vi "Refactor Object for Library Rename.vi"(8 "error in (no error)":errorcluster, 10 "rename data":T2, 11 "object reference in":refnum<vi>) -> (0 "error out":errorcluster, 1 "refactored dependency":bool, 2 "refactor result":T1, 3 "object reference out":refnum<vi>)   [LabVIEW 2020, in "MeasurementService Editor.lvlib"]
uses:
  MeasurementService Editor.lvlib
  Rename Refactor Data.ctl
  Rename Refactor Mapping Info.ctl
  Rename Refactor Result.ctl
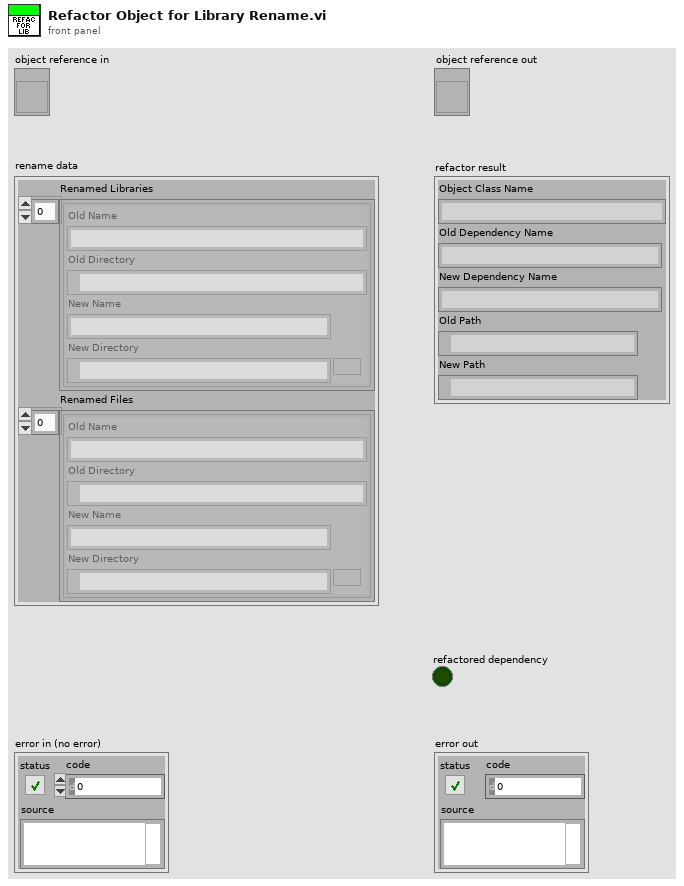
[diagram p1: front panel]
types:
  T1 = typedef "MeasurementService Editor.lvlib/Rename Refactor Result.ctl" = cluster{"Object Class Name":string, "Old Dependency Name":string, "New Dependency Name":string, "Old Path":path, "New Path":path}
  T2 = typedef "MeasurementService Editor.lvlib/Rename Refactor Data.ctl" = cluster{"Renamed Libraries":T3[], "Renamed Files":T3[]}
  T3 = typedef "MeasurementService Editor.lvlib/Rename Refactor Mapping Info.ctl" = cluster{"Old Name":string, "Old Directory":path, "New Name":string, "New Directory":path}
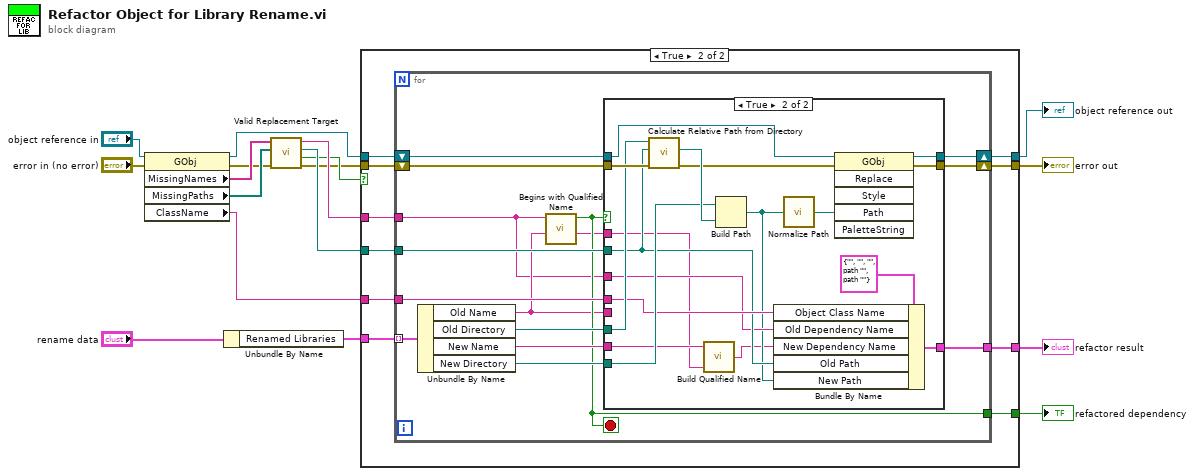
[diagram p0: block diagram]
diagram:
  n1 = property class="GObj"(reference="object reference in", error in="error in (no error)") -> (reference out=w8:refnum<vi>, error out=w2:errorcluster, "MissingNames"=w7:string[], "MissingPaths"=w6:path[], "ClassName"=w15:string)
  n2 = Unbundle By Name("rename data") -> ("Renamed Libraries"=w14:T3[])
  n3 = call "Valid Replacement Target.vi"("error in (no error)"=w2, "missing paths"=w6, "missing names"=w7) -> ("error out"=w1:errorcluster, "valid replacement target"=w3:bool, "missing path"=w4:path, "missing name"=w5:string)  [unwired: 5 in]
  n4 = case shown="True" w3 {
    tunnel: w8 -> [w18 w29]
    tunnel: w1 -> [w19 w28]
    tunnel: w5 -> [_ w20]
    tunnel: [w19 w23] -> w10
    tunnel: [w18 w24] -> w9
    tunnel: w15 -> [_ w25]
    tunnel: w4 -> [_ w26]
    tunnel: w14 -> [_ w27]
    tunnel: [_ w22] -> w12
    tunnel: [_ w21] -> w11
    frame False {
    }
    frame True {
      n5 = for {
        shift-right: [w40] -> w23
        shift-left: w28 -> [w42]
        shift-right: [w41] -> w24
        shift-left: w29 -> [w43]
        tunnel: w27 -> [w44] mode=indexing
        tunnel: w26 -> [w38]
        tunnel: [w33] -> w22
        tunnel: w25 -> [w36]
        tunnel: [w34] -> w21
        tunnel: w20 -> [w30]
        stop <- w33 stop-if-true
        n6 = Unbundle By Name(w44) -> ("Old Name"=w32:string, "Old Directory"=w39:path, "New Name"=w35:string, "New Directory"=w37:path)
        n7 = call "Begins with Qualified Name.vi"("beginning name"=w32, "name"=w30) -> ("ending name"=w31:string, "begins with name"=w33:bool)  [unwired: 8 in]
        n8 = case shown="True" w33 {
          tunnel: w43 -> [w46 w57]
          tunnel: w42 -> [w45 w64]
          tunnel: [w46 w58] -> w41
          tunnel: [w45 w60] -> w40
          tunnel: w39 -> [_ w63]
          tunnel: w38 -> [_ w54]
          tunnel: w37 -> [_ w61]
          tunnel: w36 -> [_ w55]
          tunnel: w32 -> [_ _]
          tunnel: w35 -> [_ w49]
          tunnel: [_ w53] -> w34
          tunnel: w31 -> [_ w48]
          tunnel: w30 -> [_ w52]
          frame False {
          }
          frame True {
            n9 = call "Calculate Relative Path from Directory.vi"("error in (no error)"=w64, "path"=w54, "directory"=w63) -> ("error out"=w59:errorcluster, "relative path"=w62:path)  [unwired: 7 in]
            n10 = call "Build Qualified Name.vi"("name"=w48, "base name"=w49) -> ("appended name"=w47:string)  [unwired: 3 in]
            n11 = Build Path(base path=w61, name or relative path=w62) -> (appended path=w51:path)
            n12 = Bundle By Name(cluster=T1 {"Object Class Name"="", "Old Dependency Name"="", "New Dependency Name"="", "Old Path"=path "", "New Path"=path ""} ("Rename Refactor Result"), "Object Class Name"=w55, "Old Dependency Name"=w52, "New Dependency Name"=w47, "Old Path"=w54, "New Path"=w51) -> (w53:T1)
            n13 = call "Normalize Path.vi"("path"=w51) -> ("normalized path"=w50:path)
            n14 = invoke class="GObj" method="Replace"(reference=w57, error in=w59, "Path"=w50) -> (reference out=w58:refnum<vi>, error out=w60:errorcluster)  [unwired: 3 in, 4 out]
          }
        }
      }
    }
  }
  "error out" <- w10
  "object reference out" <- w9
  "refactor result" <- w11
  "refactored dependency" <- w12
